vi "ShortcutMenu.vi"(8 "error in":errorcluster, 9 "menu ref in":refnum<k9>, 11 "node in":refnum<class "RIO Target.lvclass">) -> (0 "error out":errorcluster, 1 "menu ref out":refnum<k9>, 3 "node out":refnum<class "RIO Target.lvclass">)   [LabVIEW 2014, in "RIO Target.lvclass"]
doc: "Defines the behavior of the shortcut menu of the node."
uses:
  RIO Target.lvclass
  <vilib>/NI/Configuration Framework/serializable node/NISE_CEF_serializable node.lvclass
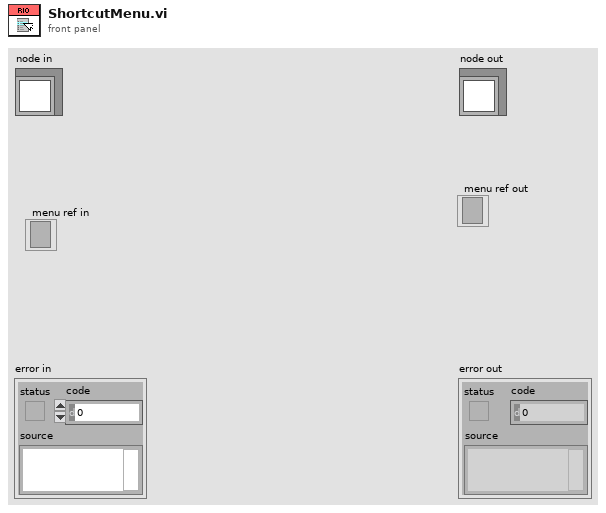
[diagram p1: front panel]
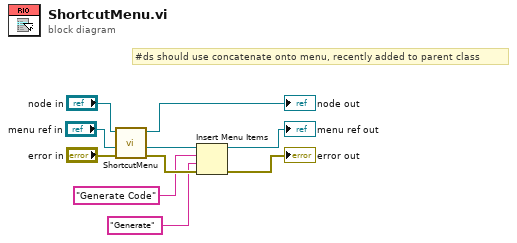
[diagram p0: block diagram]
diagram:
  # "#ds should use concatenate onto menu, recently added to parent class"
  n1 = call-parent "ShortcutMenu.vi"("error in"="error in", "menu ref in"="menu ref in", "node in"="node in") -> ("error out"=w5:errorcluster, "menu ref out"=w6:refnum<k9>, "node out"=→"node out":refnum<class "RIO Target.lvclass">)  [unwired: 6 in]
  n2 = Insert Menu Items(6:w5, 7:"Generate" ("item tags"), 8:"Generate Code", 9:w6) -> (0:→"error out":errorcluster, 3:→"menu ref out":refnum<k9>)  [unwired: 2 in, 1 out]
